vi "testTimestampParsingExplicitTimeZone.vi"(8 "error in (no error)":errorcluster, 11 "TestCase in":refnum<class "EasyXMLTest.lvclass">) -> (0 "error out":errorcluster, 3 "TestCase out":refnum<class "EasyXMLTest.lvclass">)   [LabVIEW 2013, in "EasyXMLTest.lvclass"]
doc: "Verify that error in is not overwritten"
uses:
  EasyXMLTest.lvclass
panel:
  out "dateTime out":timestamp
  out "Produced Data":variant
  out "Expected Data":variant
  out "XML String":string
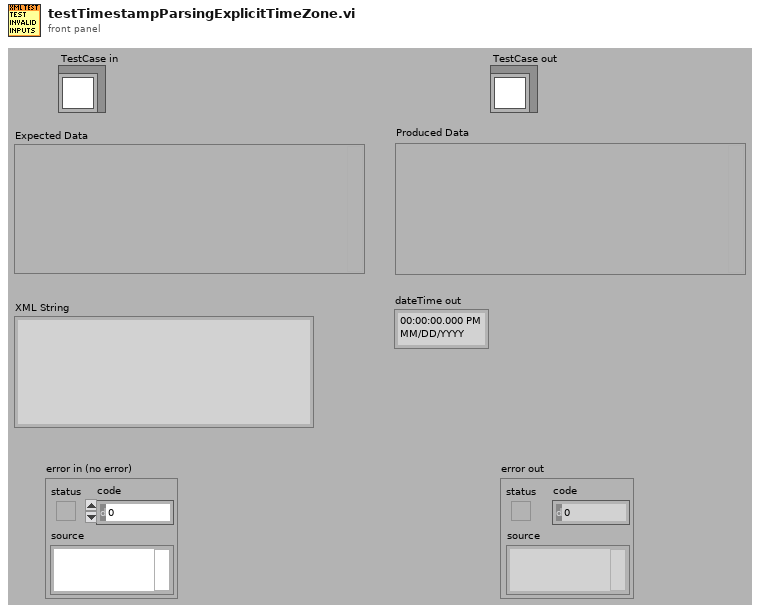
[diagram p1: front panel]
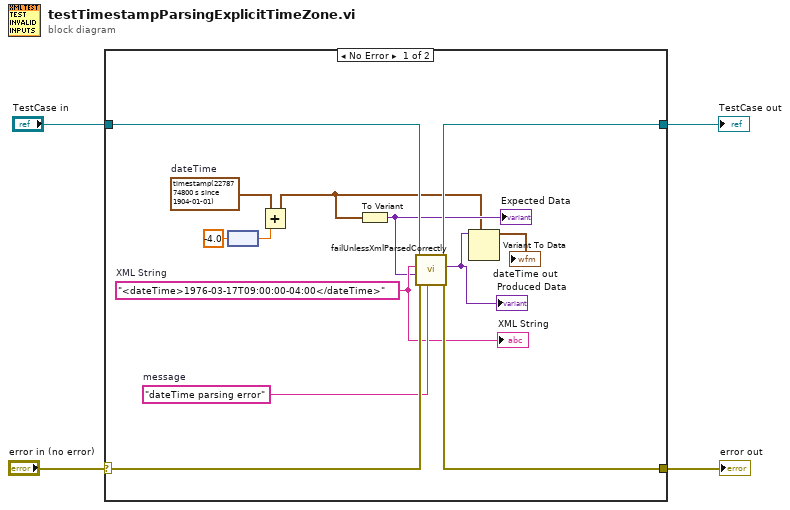
[diagram p0: block diagram]
diagram:
  n1 = case shown="No Error" "error in (no error)" {
    selector: "error in (no error)" -> [w16 w19]
    tunnel: [w15 w19] -> w2
    tunnel: [w14 w18] -> w1
    tunnel: "TestCase in" -> [w17 w18]
    frame No Error {
      w8 = timestamp(2278774800 s since 1904-01-01)  # dateTime
      w12 = "<dateTime>1976-03-17T09:00:00-04:00</dateTime>"  # XML String
      w13 = "dateTime parsing error"  # message
      n2 = node(-4.0) -> (w5:dbl[unit])
      n3 = Add(x=w8, y=w5) -> (x+y=w7:timestamp)
      n4 = To Variant(anything=w7) -> (Variant=w11:variant)
      "Expected Data" <- w11
      n5 = call "failUnlessXmlParsedCorrectly.vi"("message (\"\")"=w13, "error in"=w16, "Expected Data"=w11, "XML String"=w12, "reference in"=w17) -> ("error out"=w15:errorcluster, "Produced Data"=w10:variant, "reference in"=w14:refnum<class "EasyXMLTest.lvclass">)  [unwired: 4 in]
      "Produced Data" <- w10
      n6 = Variant To Data(type=w7, Variant=w10) -> (data=→"dateTime out":timestamp)  [unwired: 1 in, 1 out]
      "XML String" <- w12
    }
    frame Error {
    }
  }
  "error out" <- w2
  "TestCase out" <- w1
